vi "Trajectory Adaptation Algorithm_v1.vi"(0 "start (xi,yi)":dbl[](array[numeric])=[0.0, 5.0] format="%.2f", 1 "current (x,y)":dbl[](array[numeric])=[0.0, 5.0] format="%.2f", 5 "(Reye,Rassign)":dbl[](array[numeric])=[5.0, 1.0], 7 "Tassign":dbl[](array[numeric])=[0.0, 5.0], 9 "Tt":dbl, 11 "Th":dbl, 12 "index":i32) -> (4 "adaptive (x,y)":dbl[](array[numeric]), 15 "adatation over":bool)   [LabVIEW 2010]
doc: "This VI transforms the current (x,y) into a new location based on the assigned radius R assign and assigned translation vector Tassign. The location is index/time dependent: the frist Tt seconds, rotation matrix and translation vector ramp up linearly, and then it would stay for another Th seconds, after that they ramp down to what they originally were and stay there unless otherwise told to."
uses:
  <vilib>/Analysis/NI_AALBase.lvlib
  <vilib>/Analysis/baseanly.llb/A x Vector.vi
  <vilib>/Analysis/Matrix/NI_Matrix.lvlib
  <vilib>/Analysis/Matrix/Numeric/Conversions/Array To Matrix - RA2.vi
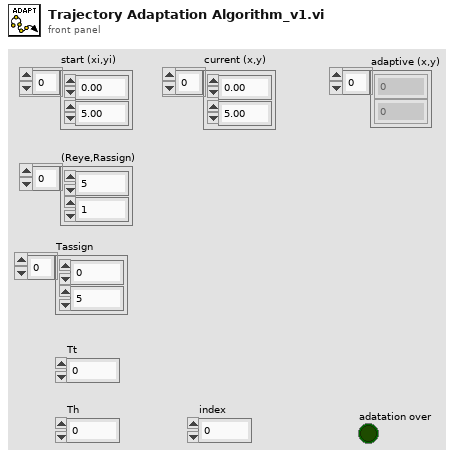
[diagram p1: front panel]
types:
  T1 = typedef "NI_Matrix.lvlib/RealMatrix.ctl" = dbl[][]
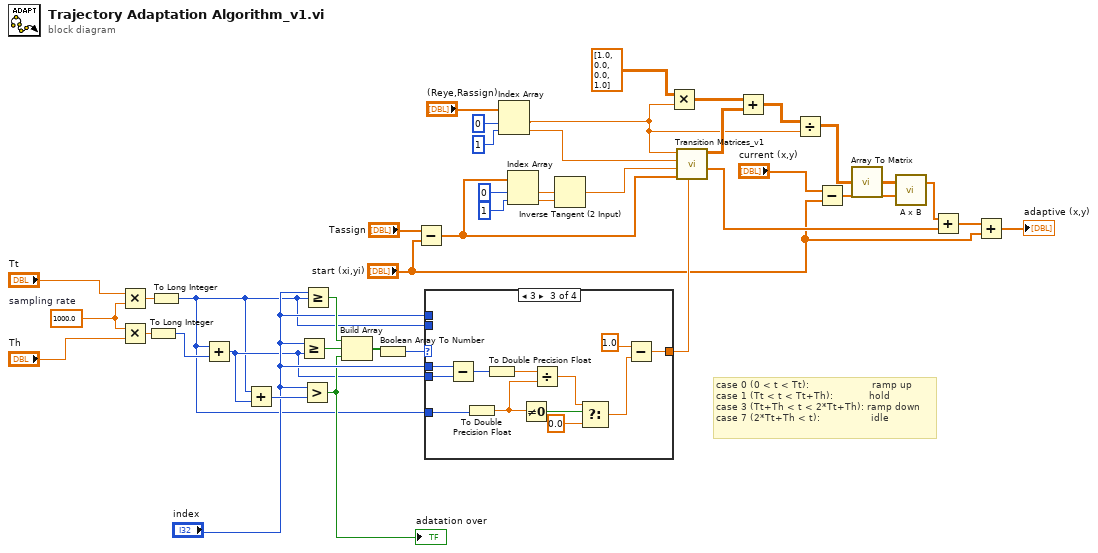
[diagram p0: block diagram]
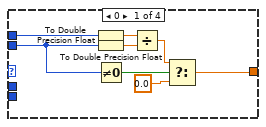
[diagram p2: hidden frame]
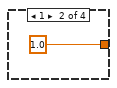
[diagram p3: hidden frame]
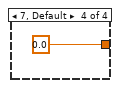
[diagram p4: hidden frame]
diagram:
  w38 = 1000.0  # sampling rate
  # "case 0 (0 < t < Tt):                     ramp up\ncase 1 (Tt < t < Tt+Th):            hold\ncase 3 (Tt+Th < t < 2*Tt+Th): ramp down\ncase 7 (2*Tt+Th < t):                 idle"
  n1 = Multiply(x="Tt", y=w38) -> (x*y=w40:dbl)
  n2 = Multiply(x=w38, y="Th") -> (x*y=w41:dbl)
  n3 = To Long Integer(number=w41) -> (32bit integer=w39:i32)
  n4 = To Long Integer(number=w40) -> (32bit integer=w1:i32)
  n5 = Add(x=w1, y=w39) -> (x+y=w2:i32)
  n6 = Add(x=w1, y=w2) -> (x+y=w31:i32)
  n7 = Greater Or Equal?(x="index", y=w2) -> (x >= y?=w34:bool)
  n8 = Greater?(x="index", y=w31) -> (0:w3:bool)
  "adatation over" <- w3
  n9 = Greater Or Equal?(x="index", y=w1) -> (x >= y?=w35:bool)
  n10 = Build Array(w35, w34, w3) -> (w33:bool[])
  n11 = Boolean Array To Number(Boolean array=w33) -> (number=w32:u32)
  n12 = Subtract(x="Tassign", y="start (xi,yi)") -> (x-y=w8:dbl[])
  n13 = case shown="3" w32 {
    tunnel: w1 -> [w46 _ _ _]
    tunnel: "index" -> [w47 _ _ _]
    tunnel: [w43 1.0 w59 0.0] -> w30
    tunnel: "index" -> [_ _ w61 _]
    tunnel: w2 -> [_ _ w60 _]
    tunnel: w1 -> [_ _ w56 _]
    frame 0 {
      n14 = To Double Precision Float(number=w47) -> (double precision float=w49:dbl)
      n15 = To Double Precision Float(number=w46) -> (double precision float=w48:dbl)
      n16 = Not Equal To 0?(x=w46) -> (x != 0?=w45:bool)
      n17 = Divide(x=w49, y=w48) -> (x/y=w44:dbl)
      n18 = Select(t=w44, s=w45, f=0.0) -> (s? t:f=w43:dbl)
    }
    frame 1 {
    }
    frame 3 {
      n19 = Subtract(x=w61, y=w60) -> (x-y=w58:i32)
      n20 = To Double Precision Float(number=w56) -> (double precision float=w53:dbl)
      n21 = To Double Precision Float(number=w58) -> (double precision float=w57:dbl)
      n22 = Not Equal To 0?(x=w53) -> (x != 0?=w55:bool)
      n23 = Divide(x=w57, y=w53) -> (x/y=w51:dbl)
      n24 = Select(t=w51, s=w55, f=0.0) -> (s? t:f=w52:dbl)
      n25 = Subtract(x=1.0, y=w52) -> (x-y=w59:dbl)
    }
    frame 7, Default {
    }
  }
  n26 = Index Array(array="(Reye,Rassign)", index #1=0 ("index"), index #2=1 ("index")) -> (element #1=w10:dbl, element #2=w9:dbl)
  n27 = Index Array(array=w8, index #1=0 ("index"), index #2=1 ("index")) -> (element #1=w25:dbl, element #2=w24:dbl)
  n28 = Inverse Tangent (2 Input)(1:w24, 2:w25) -> (0:w23:dbl)
  n29 = Multiply(x=dbl[][] [[1.0, 0.0], [0.0, 1.0]], y=w10) -> (x*y=w21:dbl[][])
  n30 = call "Transition Matrices_v1.vi"("alpha"=w30, "Tassign"=w8, "theta"=w23, "Rassign"=w9, "R0"=w10) -> ("Translation Vector"=w36:dbl[], "Rotation Matrix"=w37:dbl[][])  [unwired: 5 in]
  n31 = Add(x=w21, y=w37) -> (x+y=w28:dbl[][])
  n32 = Divide(x=w28, y=w10) -> (x/y=w19:dbl[][])
  n33 = Subtract(x="current (x,y)", y="start (xi,yi)") -> (x-y=w16:dbl[])
  n34 = call-poly <vilib>:"Array To Matrix.vi"("Real 2D Array"=w19) -> ("Real Matrix"=w20:T1)
  n35 = call-poly <vilib>:"A x B.vi"("Vector"=w16, "A"=w20) -> ("A x Vector"=w29:dbl[])  [unwired: 1 out]
  n36 = Add(x=w29, y=w36) -> (x+y=w15:dbl[])
  n37 = Add(x=w15, y="start (xi,yi)") -> (x+y=→"adaptive (x,y)":dbl[])
